vi "Measure Single Point With Compliance.vi"(8 "error in (no error)":errorcluster, 11 "KeysightDmm in":refnum<class "KeysightDmm.lvclass">) -> (0 "error out":errorcluster, 1 "Out_Of_Range":bool, 2 "Measured_Value":dbl, 3 "KeysightDmm out":refnum<class "KeysightDmm.lvclass">)   [LabVIEW 2021, in "KeysightDmm.lvclass"]
uses:
  KeysightDmm.lvclass
  KeysightDmm.lvclass/KeysightDmm.ctl
  <instrlib>/Agilent 34401/Public/Data/Read (Single Point).vi
  <instrlib>/Agilent 34401/Agilent 34401.lvlib
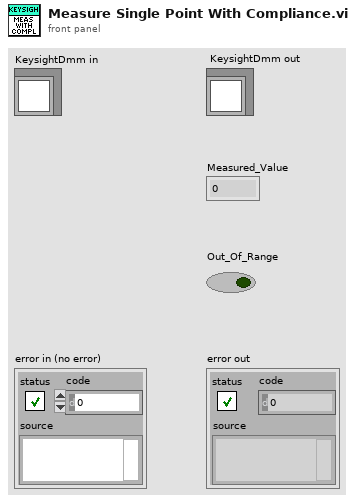
[diagram p1: front panel]
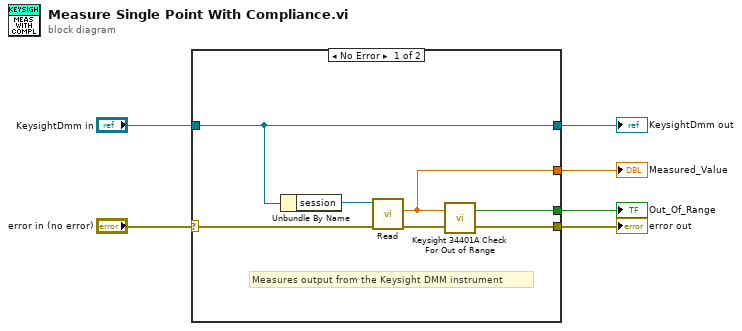
[diagram p0: block diagram]
diagram:
  n1 = case shown="No Error" "error in (no error)" {
    selector: "error in (no error)" -> [w12 w13]
    tunnel: [w11 w13] -> w5
    tunnel: "KeysightDmm in" -> [w9 w14]
    tunnel: [w9 w14] -> w3
    tunnel: [w8 _] -> w2
    tunnel: [w7 _] -> w1
    frame No Error {
      # "Measures output from the Keysight DMM instrument"
      n2 = Unbundle By Name(w9) -> ("session"=w10:refnum<visa-resource-name>)
      n3 = call-poly <instrlib>:"Read.vi"("error in (no error)"=w12, "VISA resource name"=w10) -> ("error out"=w11:errorcluster, "Measurement"=w8:dbl)  [unwired: 7 in, 1 out]
      n4 = call "Keysight 34401A Check For Out of Range.vi"("value"=w8) -> ("out of range?"=w7:bool)  [unwired: 2 in]
    }
    frame Error {
    }
  }
  "error out" <- w5
  "KeysightDmm out" <- w3
  "Measured_Value" <- w2
  "Out_Of_Range" <- w1
